vi "Dialog_Arrow Key Handler_ACAF.vi"(8 "error in (no error)":errorcluster, 10 "String Ref":refnum<vi>, 11 "Tree Ref":refnum<vi>) -> (0 "error out":errorcluster)   [LabVIEW 2023]
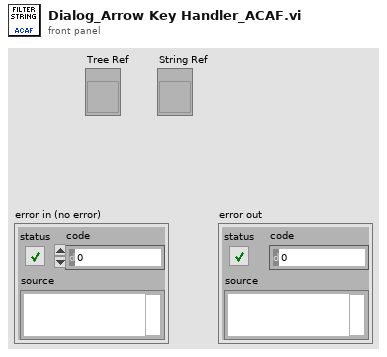
[diagram p1: front panel]
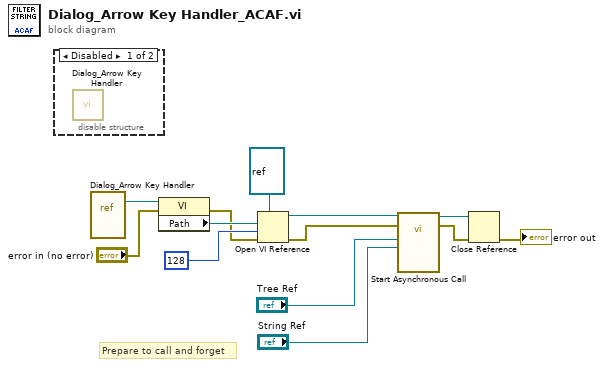
[diagram p0: block diagram]
diagram:
  # "Prepare to call and forget"
  n1 = disable-structure shown="Disabled" {
    frame Disabled {
      n2 = call "Dialog_Arrow Key Handler.vi"() -> ()  [unwired: 12 in]
    }
    frame Enabled {
    }
  }
  n3 = vi-ref "Dialog_Arrow Key Handler.vi"() -> (w13:refnum<vi>)
  n4 = property class="VI"(reference=w13, error in="error in (no error)") -> (error out=w3:errorcluster, "Path"=w9:path)  [unwired: 1 out]
  n5 = Open VI Reference(type specifier VI Refnum (for type only)=refnum<vi> refnum, vi path=w9, options=128, error in (no error)=w3) -> (vi reference=w4:refnum<vi>, error out=w8:errorcluster)  [unwired: 2 in]
  n6 = call-by-ref "Start Asynchronous Call"(reference=w4, error in=w8, "String Ref"="String Ref", "Tree Ref"="Tree Ref") -> (reference out=w7:refnum<vi>, error out=w6:errorcluster)  [unwired: 10 in]
  n7 = Close Reference(reference=w7, error in (no error)=w6) -> (error out=→"error out":errorcluster)
